vi "getMessage.vi"(8 "error in (no error)":errorcluster, 11 "SerialClient in":refnum<class "SerialCommunication.lvclass">) -> (0 "error out":errorcluster, 2 "String":string, 3 "SerialClient out":refnum<class "SerialCommunication.lvclass">)   [LabVIEW 2016, in "SerialCommunication.lvclass"]
uses:
  SerialCommunication.lvclass
  SerialCommunication.lvclass/SerialCommunication.ctl
  common_serialprotocols/SerialCommunicator/SerialCommunicator.lvclass
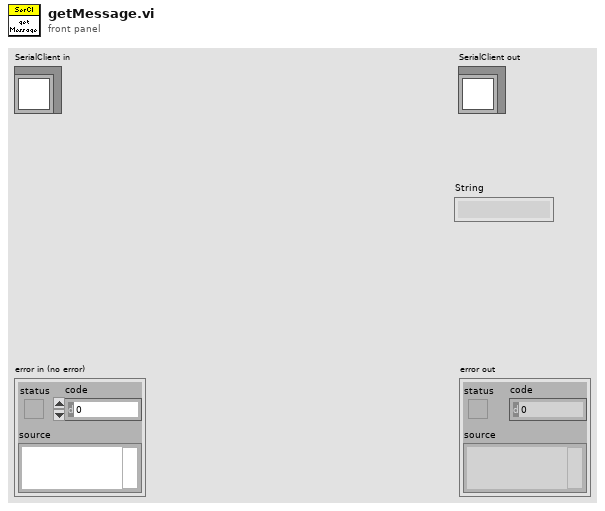
[diagram p1: front panel]
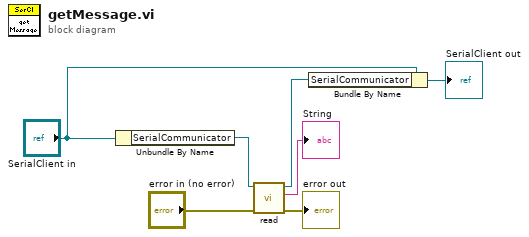
[diagram p0: block diagram]
diagram:
  n1 = Unbundle By Name("SerialClient in") -> ("SerialCommunicator"=w4:refnum<class "SerialCommunicator.lvclass">)
  n2 = call-dynamic "read.vi"("error in (no error)"="error in (no error)", "SerialCommunicator in"=w4) -> ("error out"=→"error out":errorcluster, "stringRead"=→"String":string, "SerialCommunicator out"=w2:refnum<class "SerialCommunicator.lvclass">)  [unwired: 7 in]
  n3 = Bundle By Name(cluster="SerialClient in", "SerialCommunicator"=w2) -> (→"SerialClient out":refnum<class "SerialCommunication.lvclass">)
